vi "CD Config Settings FG.vi"(6 "Action":T2, 7 "UI Refs":T1, 8 "Error In":errorcluster, 9 "Force":bool, 10 "CD Settings in":T3={"CD Task Dependency"=18446744073709551615, "CD Task Dependency Ref"=18446744073709551615, "CD Task Available Wfms"=[], "CD Task Selected Wfms"=[], "Buffer Length (samples)"=0, "Min Enabled"=FALSE, "Max Enabled "=FALSE, "SP Enabled"=FALSE, "RMS Enabled"=FALSE, "Buffer Length (s)"=0.0, "Task Rate"=0.0, "Number of DAQ Chanels"=0} {"CD Task Dependency Ref" format="%.0x"; "CD Task Dependency" format="%.0x"}, 11 "Item Ref":T4 format="%.0x") -> (0 "Error Out":errorcluster, 2 "CD Settings out":T3={"CD Task Dependency"=18446744073709551615, "CD Task Dependency Ref"=18446744073709551615, "CD Task Available Wfms"=[], "CD Task Selected Wfms"=[], "Buffer Length (samples)"=0, "Min Enabled"=FALSE, "Max Enabled "=FALSE, "SP Enabled"=FALSE, "RMS Enabled"=FALSE, "Buffer Length (s)"=0.0, "Task Rate"=0.0, "Number of DAQ Chanels"=0} {"CD Task Dependency Ref" format="%.0x"; "CD Task Dependency" format="%.0x"}, 3 "Item Ref out":T4=18446744073709551615 format="%.0x", 5 "UI Refs out":T1)   [LabVIEW 2017, in "Waveform-Processing-Custom-Device Shared.lvlib"]
doc: "This application will either \"Get\" or \"Set\" the current settings into the VeriStand system settings \nThe Set function will update or alter the VeriStand settings\nThe Get will retrieve the data from the VeriStand settings"
uses:
  Waveform-Processing-Custom-Device Shared.lvlib
  <vilib>/NI Veristand/Custom Device API/Custom Device Item Ref.ctl
  Custom Device Settings.ctl
  Types/FG Action.ctl
  System Explorer/Types/UI Refs Ctl.ctl
  Constants.vi
  <vilib>/NI Veristand/Custom Device API/Get Item Property (Dependent Node Pointer).vi
  <vilib>/NI Veristand/Custom Device API/Get Item Property (String Array).vi
  <vilib>/NI Veristand/Custom Device API/Get Item Property (U32).vi
  <vilib>/NI Veristand/Custom Device API/Get Item Property (Boolean).vi
  <vilib>/NI Veristand/Custom Device API/Get Item Property (Double).vi
  <vilib>/NI Veristand/Custom Device API/Set Item Property (Dependent Node Pointer).vi
  <vilib>/NI Veristand/Custom Device API/Set Item Property (String Array).vi
  <vilib>/NI Veristand/Custom Device API/Set Item Property (U32).vi
  <vilib>/NI Veristand/Custom Device API/Set Item Property (Boolean).vi
  <vilib>/NI Veristand/Custom Device API/Set Item Property (Double).vi
  <vilib>/NI VeriStand/Custom Device API/Custom Device API.lvlib
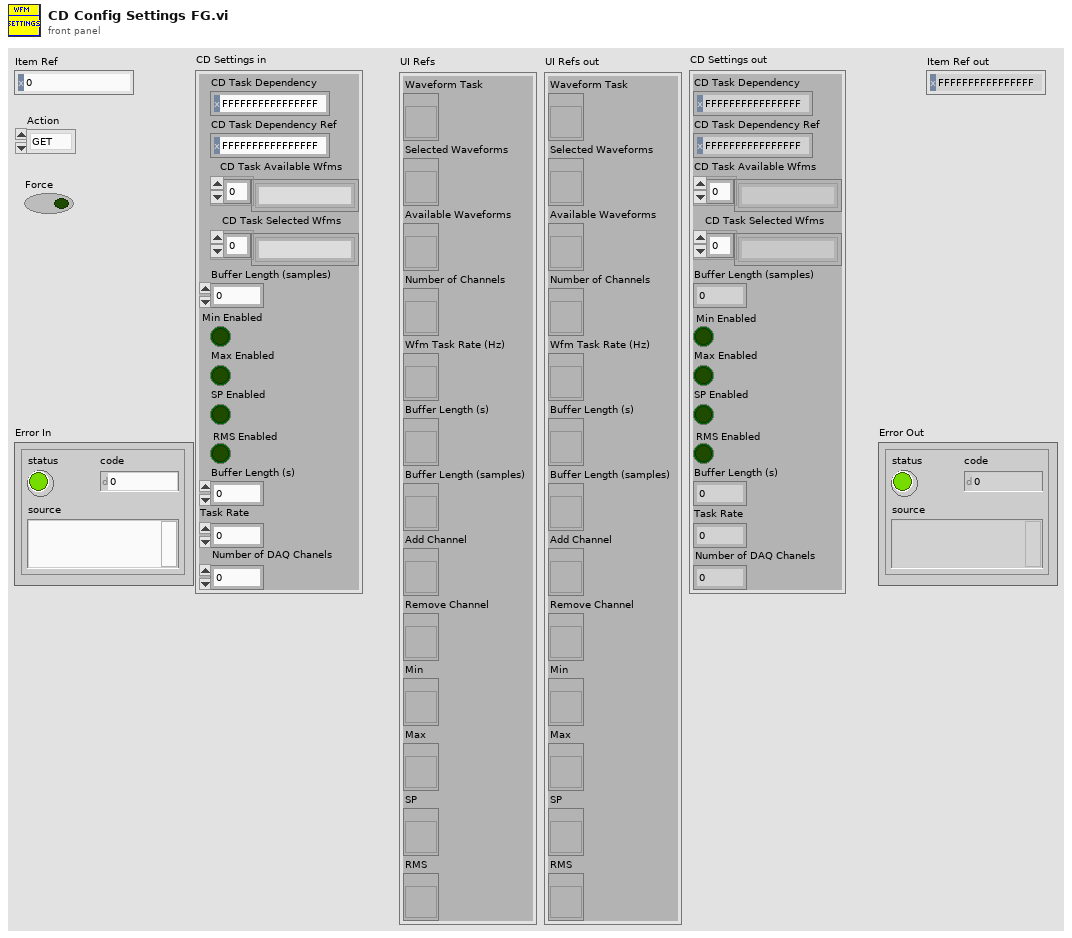
[diagram p1: front panel]
types:
  T1 = typedef "Waveform-Processing-Custom-Device Shared.lvlib/UI Refs Ctl.ctl" = cluster{"Waveform Task":refnum<vi>, "Selected Waveforms":refnum<vi>, "Available Waveforms":refnum<vi>, "Number of Channels":refnum<vi>, "Wfm Task Rate (Hz)":refnum<vi>, "Buffer Length (s)":refnum<vi>, "Buffer Length (samples)":refnum<vi>, "Add Channel":refnum<vi>, "Remove Channel":refnum<vi>, "Min":refnum<vi>, "Max":refnum<vi>, "SP":refnum<vi>, "RMS":refnum<vi>}
  T2 = typedef "Waveform-Processing-Custom-Device Shared.lvlib/FG Action.ctl" = enum8{"GET", "SET"}
  T3 = typedef "Waveform-Processing-Custom-Device Shared.lvlib/Custom Device Settings.ctl" = cluster{"CD Task Dependency":T4, "CD Task Dependency Ref":T4, "CD Task Available Wfms":string[], "CD Task Selected Wfms":string[], "Buffer Length (samples)":u32, "Min Enabled":bool, "Max Enabled ":bool, "SP Enabled":bool, "RMS Enabled":bool, "Buffer Length (s)":dbl, "Task Rate":dbl, "Number of DAQ Chanels":u32}
  T4 = typedef "Custom Device API.lvlib/Custom Device Item Ref.ctl" = u64
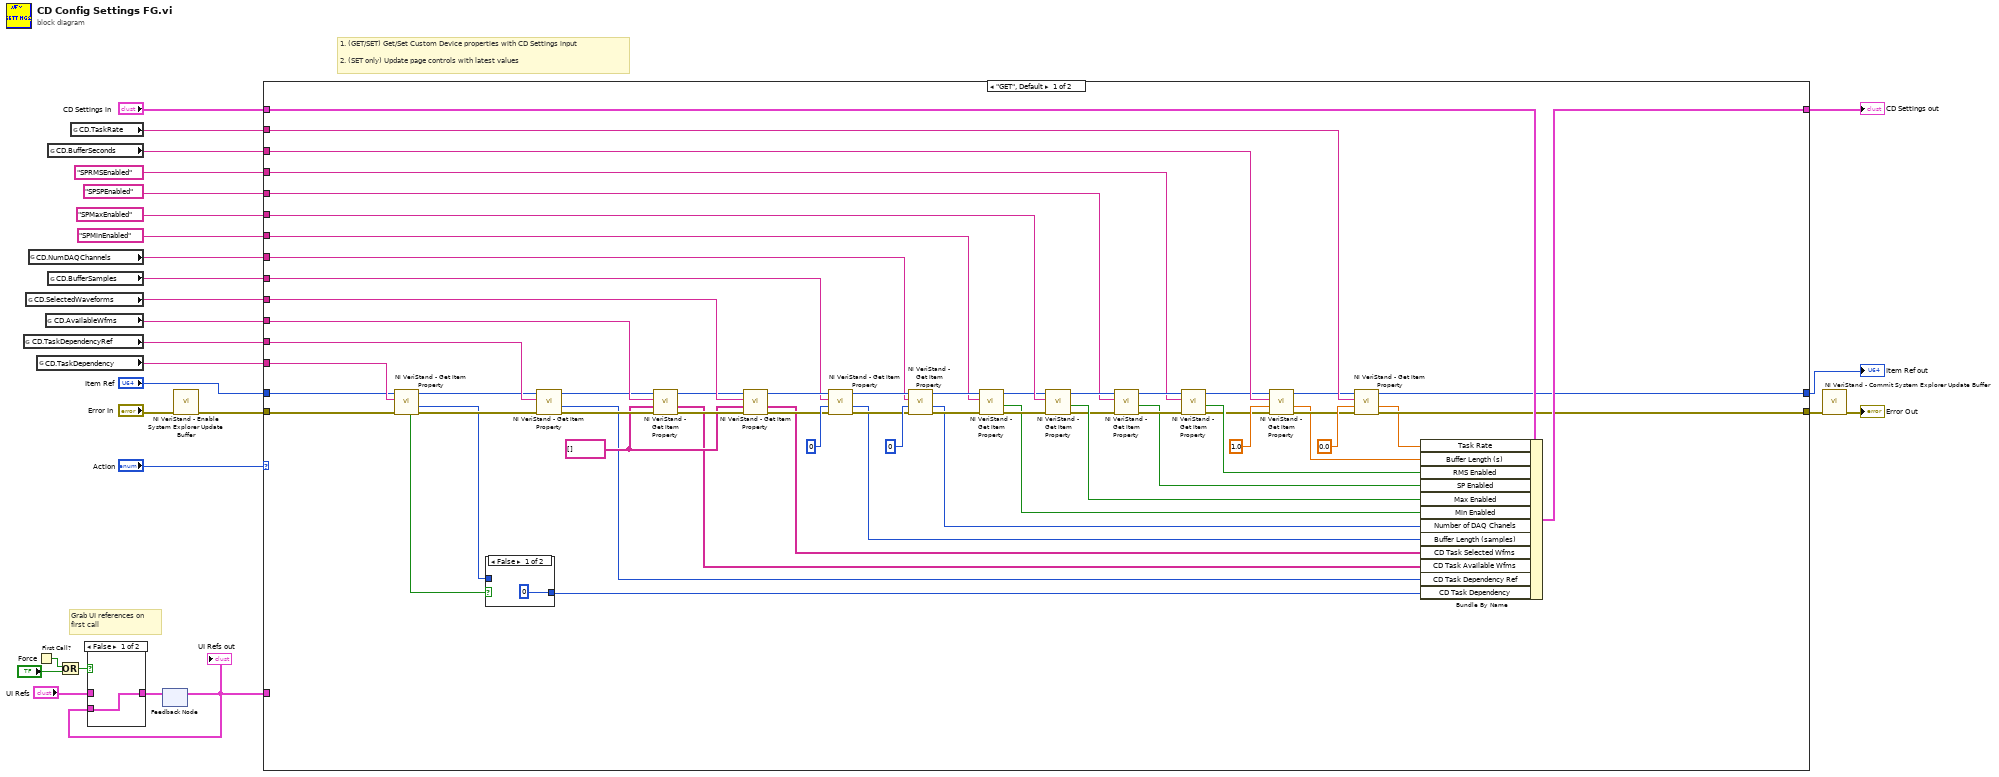
[diagram p0: block diagram]
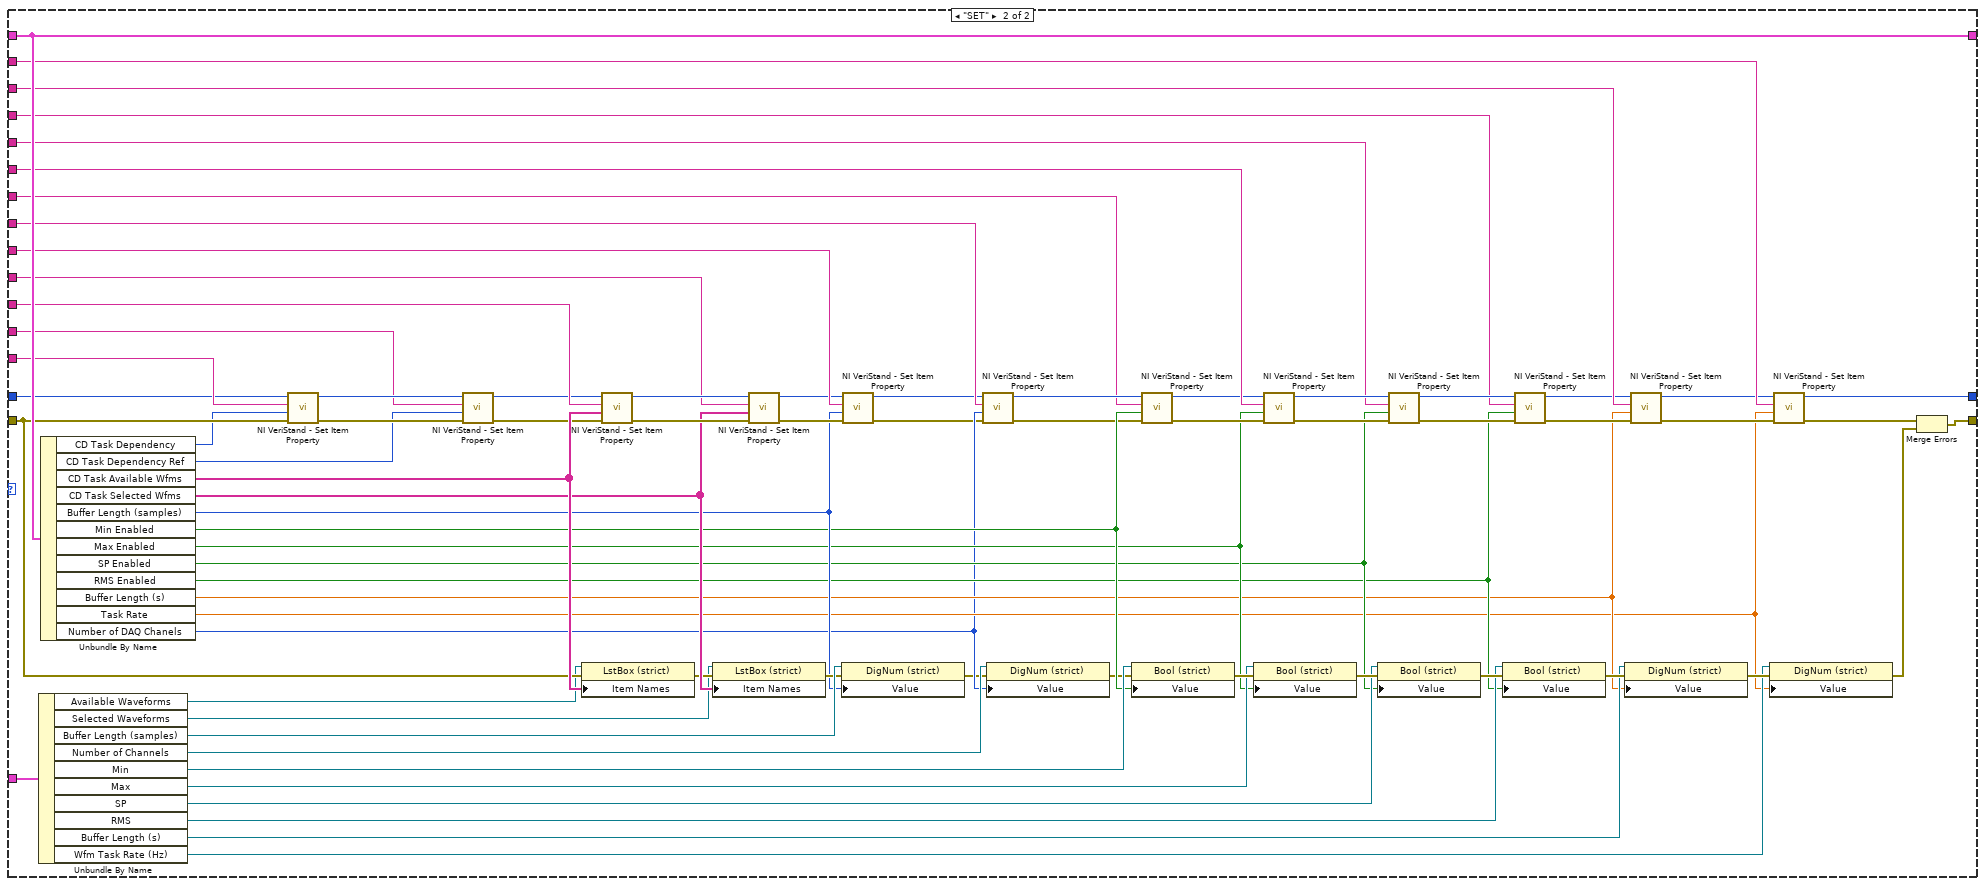
[diagram p3: hidden frame]
diagram:
  # "Grab UI references on\nfirst call"
  # "1. (GET/SET) Get/Set Custom Device properties with CD Settings input\n\n2. (SET only) Update page controls with latest values"
  n1 = global read "Constants.vi" "CD.TaskDependencyRef"() -> (w26:string)
  n2 = global read "Constants.vi" "CD.SelectedWaveforms"() -> (w24:string)
  n3 = global read "Constants.vi" "CD.NumDAQChannels"() -> (w7:string)
  n4 = First Call?() -> (First Call?: T/F=w9:bool)
  n5 = global read "Constants.vi" "CD.TaskDependency"() -> (w27:string)
  n6 = global read "Constants.vi" "CD.AvailableWfms"() -> (w25:string)
  n7 = global read "Constants.vi" "CD.BufferSeconds"() -> (w14:string)
  n8 = global read "Constants.vi" "CD.BufferSamples"() -> (w6:string)
  n9 = Or(x=w9, y="Force") -> (x .or. y?=w10:bool)
  n10 = global read "Constants.vi" "CD.TaskRate"() -> (w13:string)
  n11 = feedback #1() -> (w15:T1)  [unwired: 1 in]
  "UI Refs out" <- w15
  n12 = case shown="False" w10 {
    tunnel: "UI Refs" -> [_ w29]
    tunnel: [w28 w29] -> w17
    tunnel: w15 -> [w28 _]
    frame False {
    }
    frame True {
    }
  }
  n13 = feedback-in #1(w17) -> ()
  n14 = call <vilib>:"NI VeriStand - Enable System Explorer Update Buffer.vi"("error in (no error)"="Error In") -> ("error out"=w21:errorcluster)  [unwired: 10 in]
  n15 = case shown="\"GET\", Default" "Action" {
    tunnel: w21 -> [w56 w137]
    tunnel: "Item Ref" -> [w57 w138]
    tunnel: "CD Settings in" -> [w74 w163]
    tunnel: w27 -> [w88 w161]
    tunnel: w26 -> [w86 w159]
    tunnel: w25 -> [w84 w158]
    tunnel: w24 -> [w82 w155]
    tunnel: "SPMinEnabled" -> [w78 w91]
    tunnel: "SPMaxEnabled" -> [w76 w153]
    tunnel: [w67 w147] -> w18
    tunnel: [w66 w93] -> w19
    tunnel: [w73 w163] -> w23
    tunnel: w15 -> [_ w146]
    tunnel: w14 -> [w70 w145]
    tunnel: w13 -> [w65 w144]
    tunnel: w7 -> [w51 w115]
    tunnel: "SPSPEnabled" -> [w40 w127]
    tunnel: "SPRMSEnabled" -> [w39 w126]
    tunnel: w6 -> [w30 w112]
    frame "GET", Default {
      w61 = string[] [] ("Default Value")
      n16 = call-poly <vilib>:"NI VeriStand - Get Item Property.vi"("error in (no error)"=w56, "Property Name"=w88, "Item Ref in"=w57) -> ("error out"=w87:errorcluster, "Dependent Node Ref"=w71:T4, "Item Ref out"=w85:T4, "Found"=w72:bool)  [unwired: 5 in]
      n17 = case shown="False" w72 {
        tunnel: w71 -> [_ w90]
        tunnel: [T4 0 ("Dependent Node Ref") w90] -> w49
        frame False {
        }
        frame True {
        }
      }
      n18 = call-poly <vilib>:"NI VeriStand - Get Item Property.vi"("error in (no error)"=w87, "Property Name"=w86, "Item Ref in"=w85) -> ("error out"=w63:errorcluster, "Dependent Node Ref"=w50:T4, "Item Ref out"=w62:T4)  [unwired: 5 in, 1 out]
      n19 = call-poly <vilib>:"NI VeriStand - Get Item Property.vi"("error in (no error)"=w63, "Default Value"=w61, "Property Name"=w84, "Item Ref in"=w62) -> ("error out"=w83:errorcluster, "Value"=w53:string[], "Item Ref out"=w81:T4)  [unwired: 4 in, 1 out]
      n20 = call-poly <vilib>:"NI VeriStand - Get Item Property.vi"("error in (no error)"=w83, "Default Value"=w61, "Property Name"=w82, "Item Ref in"=w81) -> ("error out"=w54:errorcluster, "Value"=w52:string[], "Item Ref out"=w55:T4)  [unwired: 4 in, 1 out]
      n21 = call-poly <vilib>:"NI VeriStand - Get Item Property.vi"("error in (no error)"=w54, "Default Value"=u32 0, "Property Name"=w30, "Item Ref in"=w55) -> ("error out"=w58:errorcluster, "Value"=w48:u32, "Item Ref out"=w59:T4)  [unwired: 4 in, 1 out]
      n22 = call-poly <vilib>:"NI VeriStand - Get Item Property.vi"("error in (no error)"=w58, "Default Value"=u32 0, "Property Name"=w51, "Item Ref in"=w59) -> ("error out"=w80:errorcluster, "Value"=w47:u32, "Item Ref out"=w79:T4)  [unwired: 4 in, 1 out]
      n23 = call-poly <vilib>:"NI VeriStand - Get Item Property.vi"("error in (no error)"=w80, "Property Name"=w78, "Item Ref in"=w79) -> ("error out"=w77:errorcluster, "Value"=w46:bool, "Item Ref out"=w75:T4)  [unwired: 5 in, 1 out]
      n24 = call-poly <vilib>:"NI VeriStand - Get Item Property.vi"("error in (no error)"=w77, "Property Name"=w76, "Item Ref in"=w75) -> ("error out"=w42:errorcluster, "Value"=w45:bool, "Item Ref out"=w41:T4)  [unwired: 5 in, 1 out]
      n25 = call-poly <vilib>:"NI VeriStand - Get Item Property.vi"("error in (no error)"=w42, "Property Name"=w40, "Item Ref in"=w41) -> ("error out"=w43:errorcluster, "Value"=w38:bool, "Item Ref out"=w44:T4)  [unwired: 5 in, 1 out]
      n26 = call-poly <vilib>:"NI VeriStand - Get Item Property.vi"("error in (no error)"=w43, "Property Name"=w39, "Item Ref in"=w44) -> ("error out"=w34:errorcluster, "Value"=w37:bool, "Item Ref out"=w36:T4)  [unwired: 5 in, 1 out]
      n27 = call-poly <vilib>:"NI VeriStand - Get Item Property.vi"("error in (no error)"=w34, "Default Value"=1.0, "Property Name"=w70, "Item Ref in"=w36) -> ("error out"=w33:errorcluster, "Value"=w32:dbl, "Item Ref out"=w35:T4)  [unwired: 4 in, 1 out]
      n28 = call-poly <vilib>:"NI VeriStand - Get Item Property.vi"("error in (no error)"=w33, "Default Value"=0.0, "Property Name"=w65, "Item Ref in"=w35) -> ("error out"=w67:errorcluster, "Value"=w31:dbl, "Item Ref out"=w66:T4)  [unwired: 4 in, 1 out]
      n29 = Bundle By Name(cluster=w74, "Task Rate"=w31, "Buffer Length (s)"=w32, "RMS Enabled"=w37, "SP Enabled"=w38, "Max Enabled"=w45, "Min Enabled"=w46, "Number of DAQ Chanels"=w47, "Buffer Length (samples)"=w48, "CD Task Selected Wfms"=w52, "CD Task Available Wfms"=w53, "CD Task Dependency Ref"=w50, "CD Task Dependency"=w49) -> (w73:T3)
    }
    frame "SET" {
      n30 = Unbundle By Name(w146) -> ("Available Waveforms"=w123:refnum<vi>, "Selected Waveforms"=w122:refnum<vi>, "Buffer Length (samples)"=w114:refnum<vi>, "Number of Channels"=w113:refnum<vi>, "Min"=w121:refnum<vi>, "Max"=w120:refnum<vi>, "SP"=w119:refnum<vi>, "RMS"=w118:refnum<vi>, "Buffer Length (s)"=w117:refnum<vi>, "Wfm Task Rate (Hz)"=w116:refnum<vi>)
      n31 = Unbundle By Name(w163) -> ("CD Task Dependency"=w124:T4, "CD Task Dependency Ref"=w125:T4, "CD Task Available Wfms"=w151:string[], "CD Task Selected Wfms"=w150:string[], "Buffer Length (samples)"=w108:u32, "Min Enabled"=w107:bool, "Max Enabled"=w106:bool, "SP Enabled"=w105:bool, "RMS Enabled"=w104:bool, "Buffer Length (s)"=w103:dbl, "Task Rate"=w102:dbl, "Number of DAQ Chanels"=w101:u32)
      n32 = call-poly <vilib>:"NI VeriStand - Set Item Property.vi"("error in (no error)"=w137, "Dependent Node Ref"=w124, "Property Name"=w161, "Item Ref in"=w138) -> ("error out"=w162:errorcluster, "Item Ref out"=w160:T4)  [unwired: 5 in, 1 out]
      n33 = call-poly <vilib>:"NI VeriStand - Set Item Property.vi"("error in (no error)"=w162, "Dependent Node Ref"=w125, "Property Name"=w159, "Item Ref in"=w160) -> ("error out"=w139:errorcluster, "Item Ref out"=w140:T4)  [unwired: 5 in, 1 out]
      n34 = property class="LstBox (strict)"(reference=w123, error in=w137, "Item Names"=w151) -> (error out=w149:errorcluster)  [unwired: 1 out]
      n35 = call-poly <vilib>:"NI VeriStand - Set Item Property.vi"("error in (no error)"=w139, "Value"=w151, "Property Name"=w158, "Item Ref in"=w140) -> ("error out"=w157:errorcluster, "Item Ref out"=w156:T4)  [unwired: 5 in, 1 out]
      n36 = property class="LstBox (strict)"(reference=w122, error in=w149, "Item Names"=w150) -> (error out=w109:errorcluster)  [unwired: 1 out]
      n37 = call-poly <vilib>:"NI VeriStand - Set Item Property.vi"("error in (no error)"=w157, "Value"=w150, "Property Name"=w155, "Item Ref in"=w156) -> ("error out"=w110:errorcluster, "Item Ref out"=w111:T4)  [unwired: 5 in, 1 out]
      n38 = property class="DigNum (strict)"(reference=w114, error in=w109, "Value"=w108) -> (error out=w96:errorcluster)  [unwired: 1 out]
      n39 = call-poly <vilib>:"NI VeriStand - Set Item Property.vi"("error in (no error)"=w110, "Value"=w108, "Property Name"=w112, "Item Ref in"=w111) -> ("error out"=w100:errorcluster, "Item Ref out"=w98:T4)  [unwired: 5 in, 1 out]
      n40 = call-poly <vilib>:"NI VeriStand - Set Item Property.vi"("error in (no error)"=w100, "Value"=w101, "Property Name"=w115, "Item Ref in"=w98) -> ("error out"=w99:errorcluster, "Item Ref out"=w97:T4)  [unwired: 5 in, 1 out]
      n41 = property class="DigNum (strict)"(reference=w113, error in=w96, "Value"=w101) -> (error out=w95:errorcluster)  [unwired: 1 out]
      n42 = property class="Bool (strict)"(reference=w121, error in=w95, "Value"=w107) -> (error out=w148:errorcluster)  [unwired: 1 out]
      n43 = call-poly <vilib>:"NI VeriStand - Set Item Property.vi"("error in (no error)"=w99, "Value"=w107, "Property Name"=w91, "Item Ref in"=w97) -> ("error out"=w154:errorcluster, "Item Ref out"=w152:T4)  [unwired: 5 in, 1 out]
      n44 = property class="Bool (strict)"(reference=w120, error in=w148, "Value"=w106) -> (error out=w128:errorcluster)  [unwired: 1 out]
      n45 = call-poly <vilib>:"NI VeriStand - Set Item Property.vi"("error in (no error)"=w154, "Value"=w106, "Property Name"=w153, "Item Ref in"=w152) -> ("error out"=w133:errorcluster, "Item Ref out"=w134:T4)  [unwired: 5 in, 1 out]
      n46 = property class="Bool (strict)"(reference=w119, error in=w128, "Value"=w105) -> (error out=w130:errorcluster)  [unwired: 1 out]
      n47 = call-poly <vilib>:"NI VeriStand - Set Item Property.vi"("error in (no error)"=w133, "Value"=w105, "Property Name"=w127, "Item Ref in"=w134) -> ("error out"=w135:errorcluster, "Item Ref out"=w136:T4)  [unwired: 5 in, 1 out]
      n48 = property class="Bool (strict)"(reference=w118, error in=w130, "Value"=w104) -> (error out=w129:errorcluster)  [unwired: 1 out]
      n49 = call-poly <vilib>:"NI VeriStand - Set Item Property.vi"("error in (no error)"=w135, "Value"=w104, "Property Name"=w126, "Item Ref in"=w136) -> ("error out"=w131:errorcluster, "Item Ref out"=w132:T4)  [unwired: 5 in, 1 out]
      n50 = property class="DigNum (strict)"(reference=w117, error in=w129, "Value"=w103) -> (error out=w141:errorcluster)  [unwired: 1 out]
      n51 = call-poly <vilib>:"NI VeriStand - Set Item Property.vi"("error in (no error)"=w131, "Value"=w103, "Property Name"=w145, "Item Ref in"=w132) -> ("error out"=w143:errorcluster, "Item Ref out"=w142:T4)  [unwired: 5 in, 1 out]
      n52 = property class="DigNum (strict)"(reference=w116, error in=w141, "Value"=w102) -> (error out=w94:errorcluster)  [unwired: 1 out]
      n53 = call-poly <vilib>:"NI VeriStand - Set Item Property.vi"("error in (no error)"=w143, "Value"=w102, "Property Name"=w144, "Item Ref in"=w142) -> ("error out"=w92:errorcluster, "Item Ref out"=w93:T4)  [unwired: 5 in, 1 out]
      n54 = Merge Errors(w92, w94) -> (w147:errorcluster)
    }
  }
  "Item Ref out" <- w19
  "CD Settings out" <- w23
  n55 = call <vilib>:"NI VeriStand - Commit System Explorer Update Buffer.vi"("error in (no error)"=w18) -> ("error out"=→"Error Out":errorcluster)  [unwired: 10 in]
